vi "mxwScript_API_XMLTemplateName_AddTemplateID.vi"(8 "error in (no error)":errorcluster, 10 "templateID":string, 11 "absolutePath":string) -> (0 "error out":errorcluster, 3 "encoded absolutePath":string)   [LabVIEW 2020]
doc: "Tag this template with a unique name to identify it for further use."
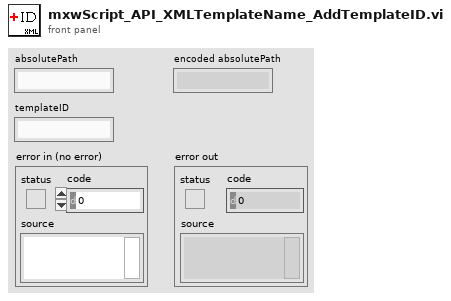
[diagram p1: front panel]
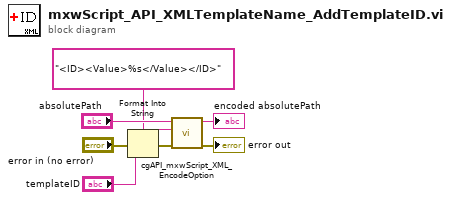
[diagram p0: block diagram]
diagram:
  n1 = Format Into String(format string="<ID><Value>%s</Value></ID>" ("control name"), error in="error in (no error)", "templateID") -> (resulting string=w2:string, error out=w4:errorcluster)  [unwired: 1 in]
  n2 = call "cgAPI_mxwScript_XML_EncodeOption.vi"("error in (no error)"=w4, "otherXML"=w2, "normalTextString"="absolutePath") -> ("error out"=→"error out":errorcluster, "encodedString"=→"encoded absolutePath":string)  [unwired: 7 out]
